vi "SDI Send Cmd.vi"(5 "CheckCRC":u8, 6 "pRespond":string, 7 "pCommand":string, 9 "SDIIndex":u8, 10 "DevIndex":i32, 11 "DevType":i32) -> (2 "function return":i32, 3 "pCommand out":string, 4 "pRespond out":string)   [LabVIEW 2010, in "ControlSDI.lvlib"]
doc: "int WINAPI SDI_SendCmd(int DevType, int DevIndex, unsigned char SDIIndex,unsigned char *pCommand,unsigned char *pRespond,unsigned char CheckCRC);"
uses:
  ControlSDI.lvlib
  ControlSDI/Ginkgo_Driver.dll
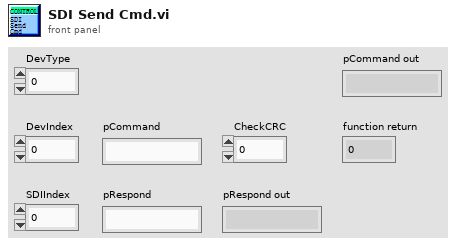
[diagram p1: front panel]
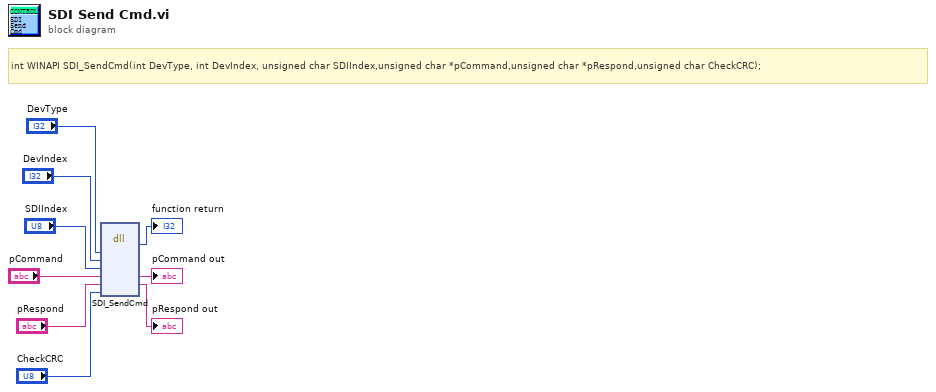
[diagram p0: block diagram]
diagram:
  # "int WINAPI SDI_SendCmd(int DevType, int DevIndex, unsigned char SDIIndex,unsigned char *pCommand,unsigned char *pRespond,unsigned char CheckCRC);"
  n1 = dll-call lib="E:/Project/vt_ginkgo/truck/Ginkgo Driver/vs2010/Ginkgo_USB-I2C&SPI&CAN_API_v2.0.3.3/lib/labview_32bit/ControlSDI/Ginkgo_Driver.*" fn="SDI_SendCmd"("DevType"="DevType", "DevIndex"="DevIndex", "SDIIndex"="SDIIndex", "pCommand"="pCommand", "pRespond"="pRespond", "CheckCRC"="CheckCRC") -> (→"function return":i32, "pCommand"=→"pCommand out":string, "pRespond"=→"pRespond out":string)  [unwired: 7 in, 2 out]
